vi "FPGA Interleaving.vi"() -> ()   [LabVIEW 2012]
panel:
  in  "stop":bool
  in  "DMA Cleared?":bool
  out "Overflow?":bool
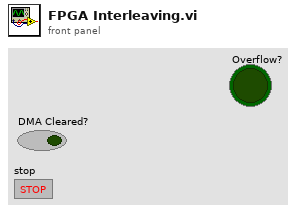
[diagram p1: front panel]
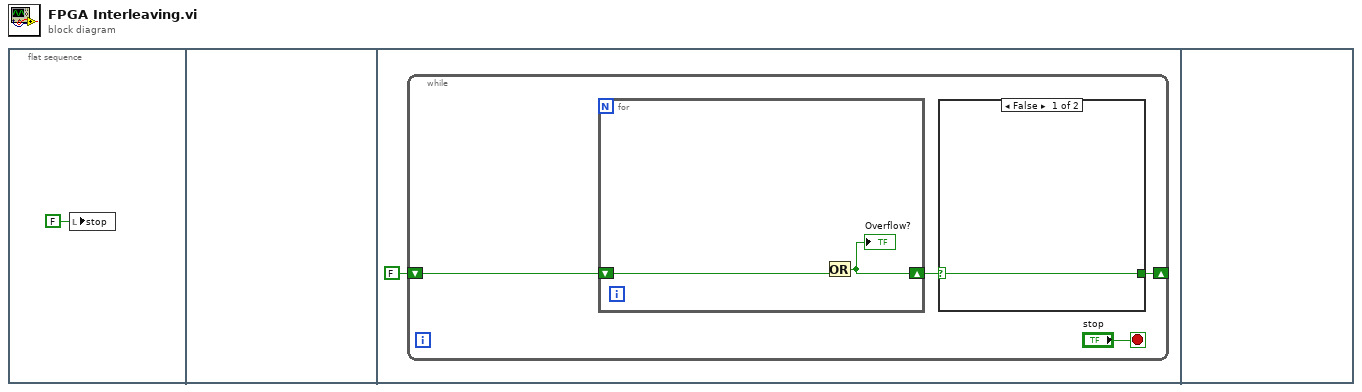
[diagram p0: block diagram]
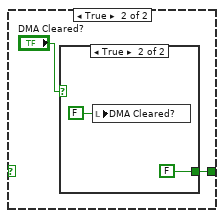
[diagram p2: hidden frame]
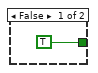
[diagram p3: hidden frame]
diagram:
  n1 = flat-sequence {
    frame #0 {
      n2 = local write "stop"(FALSE ("stop")) -> ()
    }
    frame #1 {
    }
    frame #2 {
      n3 = while {
        shift-right: [w5] -> _
        shift-left: FALSE -> [w4]
        stop <- "stop" stop-if-true
        n4 = for {
          shift-right: [w13] -> w6
          shift-left: w4 -> [w14]
          n5 = Or(y=w14) -> (x .or. y?=w13:bool)  [unwired: 1 in]
          "Overflow?" <- w13
        }
        n6 = case shown="False" w6 {
          selector: w6 -> [w7 _]
          tunnel: [w7 w8] -> w5
          frame False {
          }
          frame True {
            n7 = case shown="True" "DMA Cleared?" {
              tunnel: [TRUE FALSE] -> w8
              frame False {
              }
              frame True {
                n8 = local write "DMA Cleared?"(FALSE ("Reset")) -> ()
              }
            }
          }
        }
      }
    }
    frame #3 {
    }
  }
